vi "Build Server.vi"   [LabVIEW 2014]
uses:
  <vilib>/AppBuilder/AB_API_Simple/Build (path).vi
  <vilib>/AppBuilder/AB_API_Simple/NI_App_Builder_API.lvlib
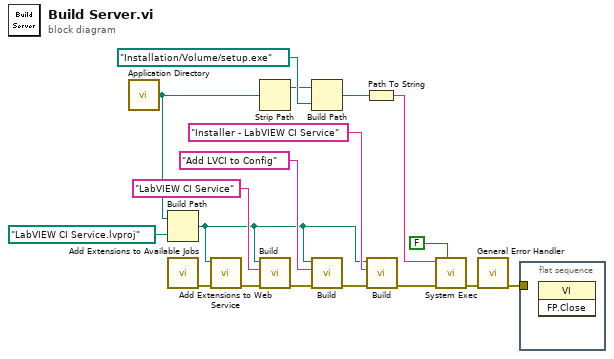
[diagram p0: block diagram]
diagram:
  n1 = call <vilib>:"Application Directory.vi"() -> ("Application Directory"=w2:path)
  n2 = Build Path(base path=w2, name or relative path=path "LabVIEW CI Service.lvproj") -> (appended path=w3:path)
  n3 = call "Add Extensions to Available Jobs.vi"() -> ("error out"=w1:errorcluster)  [unwired: 11 in]
  n4 = call "Add Extensions to Web Service.vi"("error in (no error)"=w1, "Project"=w3) -> ("error out"=w4:errorcluster)  [unwired: 9 in]
  n5 = Strip Path(path=w2) -> (stripped path=w7:path)  [unwired: 1 out]
  n6 = call-poly <vilib>:"Build.vi"("error in (no error)"=w4, "Name of build specification (if empty: build all)"="LabVIEW CI Service", "Path to project"=w3) -> ("error out"=w17:errorcluster)  [unwired: 7 in, 1 out]
  n7 = Build Path(base path=w7, name or relative path=path "Installation/Volume/setup.exe" ("Path")) -> (appended path=w9:path)
  n8 = call-poly <vilib>:"Build.vi"("error in (no error)"=w17, "Name of build specification (if empty: build all)"="Add LVCI to Config", "Path to project"=w3) -> ("error out"=w16:errorcluster)  [unwired: 7 in, 1 out]
  n9 = Path To String(path=w9) -> (string=w10:string)
  n10 = call-poly <vilib>:"Build.vi"("error in (no error)"=w16, "Name of build specification (if empty: build all)"="Installer - LabVIEW CI Service", "Path to project"=w3) -> ("error out"=w12:errorcluster)  [unwired: 7 in, 1 out]
  n11 = call <vilib>:"System Exec.vi"("wait until completion? (T)"=FALSE, "error in (no error)"=w12, "command line"=w10) -> ("error out"=w6:errorcluster)  [unwired: 5 in, 3 out]
  n12 = call <vilib>:"General Error Handler.vi"("error in (no error)"=w6) -> ("error out"=w5:errorcluster)  [unwired: 10 in, 4 out]
  n13 = flat-sequence {
    tunnel: w5 -> [_]
    frame #0 {
      n14 = invoke class="VI" method="FP.Close"() -> ()  [unwired: 3 in, 3 out]
    }
  }
